vi "LVClass_CorrectionDataManager ctor.vi"(0 "CorrectionDataManager (const)":refnum<class "CorrectionDataManager.lvclass">, 5 "PathTohaso_config_file_path":path, 7 "PathTowfc_config_file_path":path, 11 "error in (no error)":errorcluster) -> (4 "CorrectionDataManager (new)":refnum<class "CorrectionDataManager.lvclass">, 15 "error out":errorcluster)   [LabVIEW 2020, in "CorrectionDataManager.lvclass"]
doc: "CorrDataManager constructor from a Haso configuration file and a wavefront\nconfiguration file.\n\n<B>corrdata_managerIn</B> : Constant Pointer to CorrDataManager object.\n<B>corrdata_managerOut</B> : Constant Pointer to CorrDataManager object.\n<B>haso_config_file_path</B> : Absolute path to Haso configuration file.\n<B>wfc_config_file_path</B> : Absolute path to WavefrontCorrector configuration file.\n<B>use_phase</B> : use phase or slopes in correction process."
uses:
  CorrectionDataManager.lvclass
  Controls/Handle creation.ctl
  CorrectionDataManager.lvclass/CorrectionDataManager.ctl
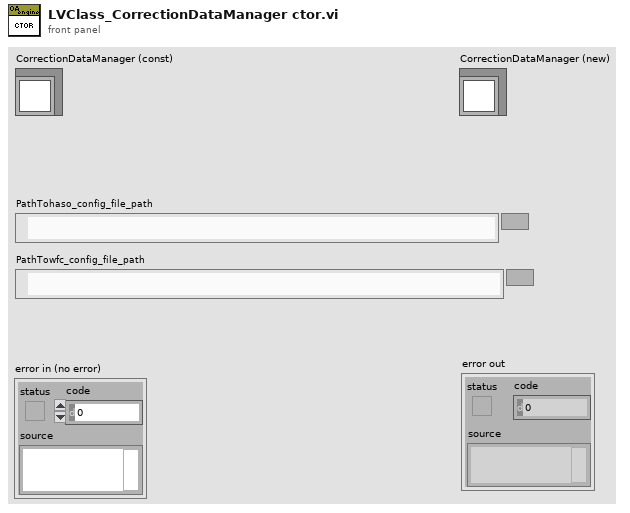
[diagram p1: front panel]
types:
  T1 = typedef "Handle creation.ctl" = enum16{"By ctor", "By write function"}
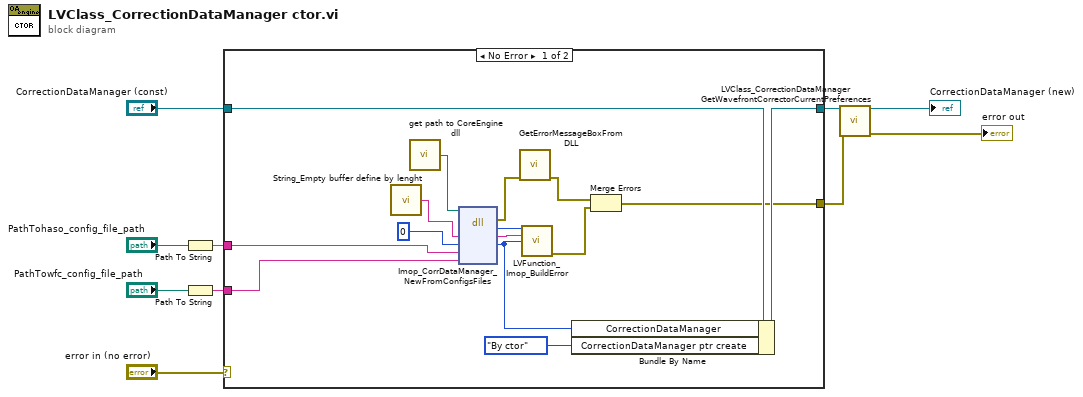
[diagram p0: block diagram]
diagram:
  n1 = Path To String(path="PathTohaso_config_file_path") -> (string=w7:string)
  n2 = Path To String(path="PathTowfc_config_file_path") -> (string=w6:string)
  n3 = case shown="No Error" "error in (no error)" {
    selector: "error in (no error)" -> [_ w27]
    tunnel: [w20 w27] -> w4
    tunnel: [w23 w26] -> w2
    tunnel: "CorrectionDataManager (const)" -> [w24 w26]
    tunnel: w7 -> [w13 _]
    tunnel: w6 -> [w12 _]
    frame No Error {
      n4 = call "String_Empty buffer define by lenght.vi"() -> ("Empty buffer"=w18:string)  [unwired: 1 in]
      n5 = call "get path to CoreEngine dll.vi"() -> ("path to wavekit library"=w19:path)  [unwired: 14 in, 1 out]
      n6 = dll-call lib="D:/soft/HASO_v3/SVN_trunk/ImOpCoreEngine4_LV2011/DLLs/c_interface_vc100.dll" fn="Imop_CorrDataManager_NewFromConfigsFiles"(path in=w19, "message"=w18, "CorrDataManager"=0 ("Pupil"), "haso_config_file_path"=w13, "wfc_config_file_path"=w12) -> (error out=w16:errorcluster, "return type"=w15:i32, "message"=w14:string, "CorrDataManager"=w11:i64)  [unwired: 4 in, 1 out]
      n7 = call "GetErrorMessageBoxFromDLL.vi"("error IN"=w16) -> ("error OUT"=w22:errorcluster)  [unwired: 10 in]
      n8 = call "LVFunction_Imop_BuildError.vi"("code"=w15, "String to Prepend to source (\"\")"=w14, "Adresse"=w11) -> ("error out"=w21:errorcluster)  [unwired: 12 in]
      n9 = Bundle By Name(cluster=w24, "CorrectionDataManager"=w11, "CorrectionDataManager ptr create"=Handle_creation."By ctor" ("Pupil ptr create")) -> (w23:refnum<class "CorrectionDataManager.lvclass">)
      n10 = Merge Errors(w22, w21) -> (w20:errorcluster)
    }
    frame Error {
    }
  }
  n11 = call "LVClass_CorrectionDataManager GetWavefrontCorrectorCurrentPreferences.vi"("CorrectionDataManager in"=w2, "error in (no error)"=w4) -> ("CorrectionDataManager out"=→"CorrectionDataManager (new)":refnum<class "CorrectionDataManager.lvclass">, "error out"=→"error out":errorcluster)  [unwired: 11 in, 1 out]
